vi "data.vi"(8 "error in (no error)":errorcluster, 11 "VISA resource name":refnum<visa-resource-name>) -> (0 "error out":errorcluster, 2 "Power":dbl, 3 "VISA resource name out":refnum<visa-resource-name>)   [LabVIEW 2009, in "Newport 1830-C.lvlib"]
doc: "AVG?=T, will return average of measurements taken 0.2 s apart for duration of averaging time.\nAVG?=F, will return one measurement.\n\nCurrent Range sets the maximum allowed value. If Power Meter reads during autoranging, will return baloney value, which this screens out and instead returns 0. Default is 10.5W for autoranging. Other ranges only work with ATTN on.\n\nWARNING! Range Query NEVER returns autoranging. If autoranging, set it manually before reading."
uses:
  Newport 1830-C.lvlib
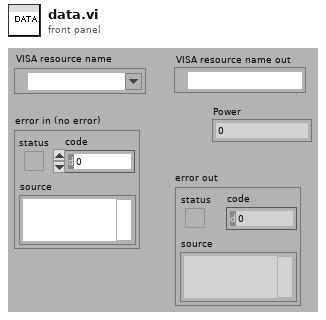
[diagram p1: front panel]
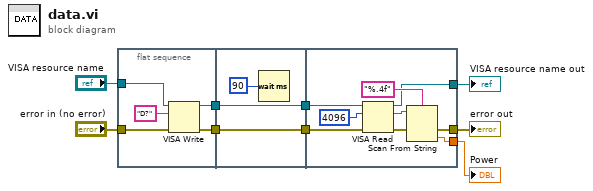
[diagram p0: block diagram]
diagram:
  n1 = flat-sequence {
    tunnel: [w13] -> w6
    tunnel: [w12] -> w5
    tunnel: "VISA resource name" -> [w11]
    tunnel: "error in (no error)" -> [w10]
    tunnel: w6 -> [w16]
    tunnel: [w17] -> w4
    tunnel: w5 -> [w17]
    tunnel: [w16] -> w3
    tunnel: w4 -> [w25]
    tunnel: w3 -> [w20]
    tunnel: [w21] -> w7
    tunnel: [w19] -> w2
    tunnel: [w18] -> w1
    frame #0 {
      n2 = VISA Write(VISA resource name=w11, write buffer="D?" ("command"), error in (no error)=w10) -> (VISA resource name out=w12:refnum<visa-resource-name>, error out=w13:errorcluster)  [unwired: 1 out]
    }
    frame #1 {
      n3 = Wait (ms)(milliseconds to wait=u32 90 ("Delay Time (s)")) -> ()  [unwired: 1 out]
    }
    frame #2 {
      n4 = VISA Read(VISA resource name=w25, byte count=u32 4096, error in (no error)=w20) -> (VISA resource name out=w21:refnum<visa-resource-name>, read buffer=w23:string, error out=w22:errorcluster)  [unwired: 1 out]
      n5 = Scan From String(format string="%.4f", input string=w23, error in=w22) -> (error out=w18:errorcluster, output 1=w19:dbl)  [unwired: 2 in, 2 out]
    }
  }
  "Power" <- w2
  "error out" <- w1
  "VISA resource name out" <- w7
